vi "SiosIfmGetRefMirrorVibrationvi.vi"(1 "Channel":i32(knob) scale=1.0..4.0, 2 "Device Number":i32) -> (0 "State of Vibration":i32)   [LabVIEW 2009]
uses:
  siosifm.dll
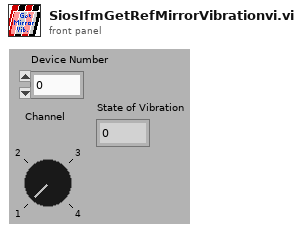
[diagram p1: front panel]
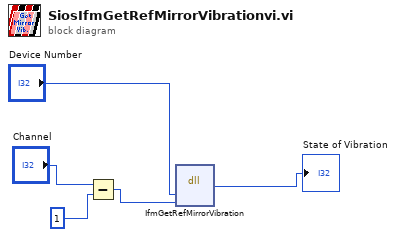
[diagram p0: block diagram]
diagram:
  n1 = Subtract(x="Channel", y=1) -> (x-y=w1:i32)
  n2 = dll-call lib="C:/WORK/Artem/RE-10/SIOS_IfmDLL/siosifm.dll" fn="IfmGetRefMirrorVibration"("devNumber"="Device Number", "channel"=w1) -> ("on_off"=→"State of Vibration":i32)  [unwired: 5 in, 2 out]
